vi "TagDB-List.vi"(8 "error in (no error)":errorcluster, 10 "with Data?(F)":bool, 11 "TagDB":T1) -> (0 "error out":errorcluster, 1 "Data":variant[](array[variant]), 2 "names":string[](array[string]), 3 "TagDB(dup)":T1)   [LabVIEW 2017, in "TagDB.lvlib"]
uses:
  TagDB.lvlib
  Typedef/TagDB.ctl
  _Support/Error/_Build Error Cluster.vi
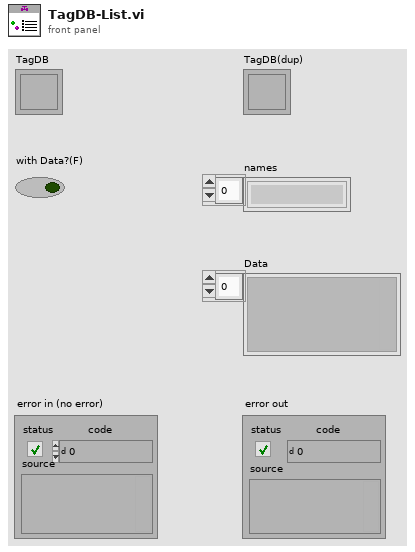
[diagram p1: front panel]
types:
  T1 = typedef "TagDB.lvlib/TagDB.ctl" = refnum<k1>
  T2 = typedef "TagDB.lvlib/tagdb-data.ctl" = cluster{"tag-map":variant, "timestamp-map":variant, "namecacher-map":variant, "DataTypeCacher-map":variant, "Tag Adding Lock?":bool, "Global Change Timestamp":timestamp, "Item Change Timestamp":timestamp, "name":string, "Global Change Flag":u64, "Item Change Flag":u64}
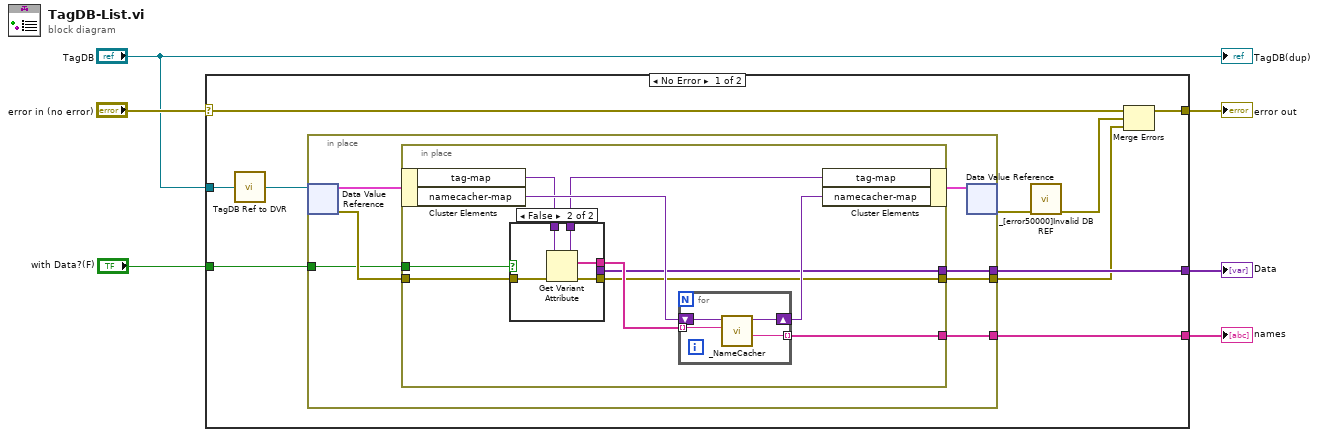
[diagram p0: block diagram]
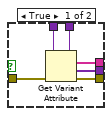
[diagram p2: hidden frame]
diagram:
  n1 = case shown="No Error" "error in (no error)" {
    selector: "error in (no error)" -> [w16 w49]
    tunnel: [w13 w49] -> w6
    tunnel: "TagDB" -> [w15 _]
    tunnel: [w11 _] -> w3
    tunnel: [w10 _] -> w2
    tunnel: "with Data?(F)" -> [w8 _]
    frame No Error {
      n2 = call "TagDB Ref to DVR.vi"("TagDB"=w15) -> ("DVR"=w14:refnum<data-value>)  [unwired: 4 in]
      n3 = in-place {
        in-place-border: [w23] -> w11
        in-place-border: [w22] -> w10
        in-place-border: [w18] -> w9
        in-place-border: w8 -> [w17]
        n4 = in-place-dvr #1(w14) -> (w21:T2, w19:errorcluster)
        n5 = in-place {
          in-place-border: [w26] -> w23
          in-place-border: [w32] -> w22
          in-place-border: w19 -> [w28]
          in-place-border: [w25] -> w18
          in-place-border: w17 -> [w24]
          n6 = in-place-cluster #2(w21) -> ("tag-map"=w30:variant, "namecacher-map"=w31:variant)
          n7 = case shown="False" w24 {
            tunnel: [w39 w44] -> w33
            tunnel: w30 -> [w38 w43]
            tunnel: [w37 w42] -> w29
            tunnel: w28 -> [w36 w41]
            tunnel: [w35 _] -> w26
            tunnel: [w34 w40] -> w25
            frame True {
              n8 = Get Variant Attribute(Variant=w38, error in=w36) -> (duplicate Variant=w37:variant, names=w39:string[], values=w35:variant[], error out=w34:errorcluster)  [unwired: 2 in]
            }
            frame False {
              n9 = Get Variant Attribute(Variant=w43, error in=w41) -> (duplicate Variant=w42:variant, names=w44:string[], error out=w40:errorcluster)  [unwired: 2 in, 1 out]
            }
          }
          n10 = for {
            tunnel: w33 -> [w48] mode=indexing
            tunnel: [w47] -> w32 mode=indexing
            shift-right: [w45] -> w27
            shift-left: w31 -> [w46]
            n11 = call "_NameCacher.vi"("key"=w48, "cacher"=w46) -> ("Raw name"=w47:string, "cacher out"=w45:variant)  [unwired: 7 in, 1 out]
          }
          n12 = in-place-cluster #2("tag-map"=w29, "namecacher-map"=w27) -> (w20:T2)
        }
        n13 = in-place-dvr #1(w20) -> (w12:errorcluster)  [unwired: 1 out]
      }
      n14 = call "_[error50000]Invalid DB REF.vi"("error in (no error)"=w12) -> ("error out"=w7:errorcluster)  [unwired: 10 in]
      n15 = Merge Errors(w16, w7, w9) -> (w13:errorcluster)
    }
    frame Error {
    }
  }
  "error out" <- w6
  "names" <- w2
  "Data" <- w3
  "TagDB(dup)" <- "TagDB"
